vi "Test Get All Elements Some Info 1.vi"() -> ()   [LabVIEW 2014]
panel:
  out "FiringOrder ClassNames":string[](array[string])
  out "elements class name and label":string[][](array[string])
  in  "vi path":path=path "C:/Users/miesizelezo/Documents/LabVIEW/LabVIEW-Universal-Transcriptor/Test/Examples For Parsing/Example FlatSequence 1.vi"
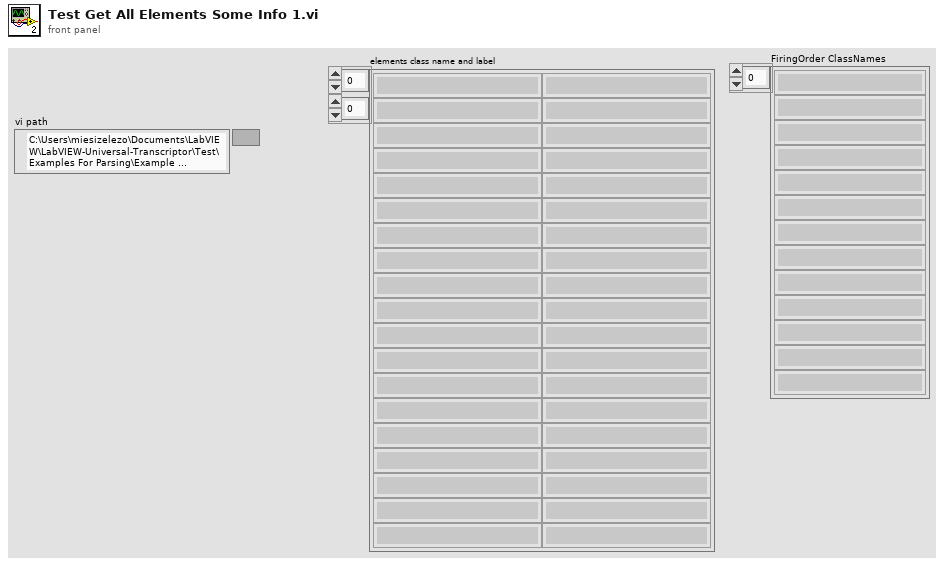
[diagram p1: front panel]
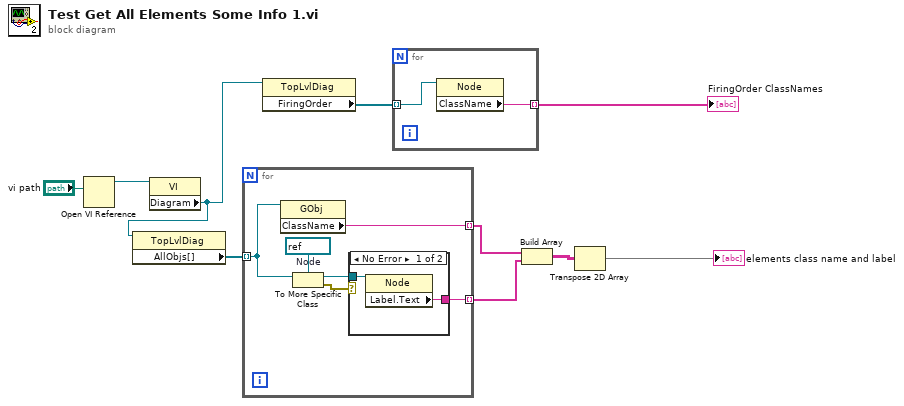
[diagram p0: block diagram]
diagram:
  n1 = Open VI Reference(vi path="vi path") -> (vi reference=w9:refnum<vi>)  [unwired: 5 in, 1 out]
  n2 = property class="VI"(reference=w9) -> ("Diagram"=w4:refnum<vi>)  [unwired: 1 in, 2 out]
  n3 = property class="TopLvlDiag"(reference=w4) -> ("AllObjs[]"=w1:refnum<vi>[])  [unwired: 1 in, 2 out]
  n4 = for {
    tunnel: w1 -> [w15] mode=indexing
    tunnel: [w16] -> w8 mode=indexing
    tunnel: [w12] -> w7 mode=indexing
    w14 = refnum<vi> refnum  # Node
    n5 = property class="GObj"(reference=w15) -> ("ClassName"=w16:string)  [unwired: 1 in, 2 out]
    n6 = To More Specific Class(target class=w14, reference=w15) -> (specific class reference=w13:refnum<vi>, error out=w11:errorcluster)  [unwired: 1 in]
    n7 = case shown="No Error" w11 {
      tunnel: w13 -> [w18 _]
      tunnel: [w17 _] -> w12
      frame No Error {
        n8 = property class="Node"(reference=w18) -> ("Label.Text"=w17:string)  [unwired: 1 in, 2 out]
      }
      frame Error {
      }
    }
  }
  n9 = property class="TopLvlDiag"(reference=w4) -> ("FiringOrder"=w3:refnum<vi>[])  [unwired: 1 in, 2 out]
  n10 = for {
    tunnel: w3 -> [w20] mode=indexing
    tunnel: [w19] -> w2 mode=indexing
    n11 = property class="Node"(reference=w20) -> ("ClassName"=w19:string)  [unwired: 1 in, 2 out]
  }
  "FiringOrder ClassNames" <- w2
  n12 = Build Array(w8, w7) -> (w6:string[][])
  n13 = Transpose 2D Array(2D array=w6) -> (transposed array=→"elements class name and label":string[][])
